vi "GetTraceFormat.vi"(8 "Error In":errorcluster, 11 "Keithley 6482 In":refnum<visa-resource-name>) -> (0 "Error Out":errorcluster, 2 "Trace Format Elements":T1[](array[typedef]), 3 "Keithley 6482 Out":refnum<visa-resource-name>)   [LabVIEW 8.6, in "Keithley-6482-Visa.lvlib"]
uses:
  Keithley-6482-Visa.lvlib
  Controls/TraceFormatElement.ctl
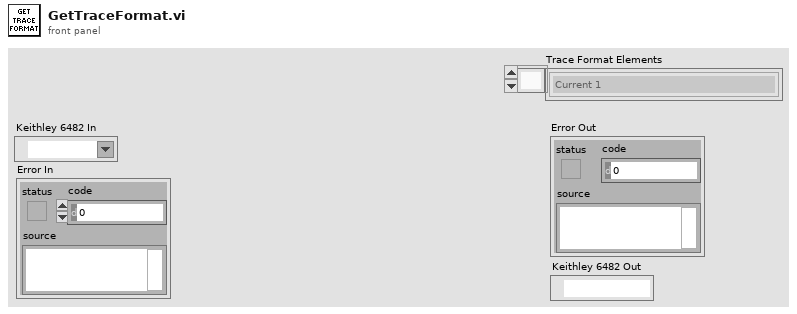
[diagram p1: front panel]
types:
  T1 = typedef "Keithley-6482-Visa.lvlib/TraceFormatElement.ctl" = enum16{"Current 1", "Current 2", "Calculate 1", "Calculate 2", "Calculate 3", "Calculate 4", "Calculate 5", "Calculate 6", "Calculate 7", "Time", "Status", "All", "Default"}
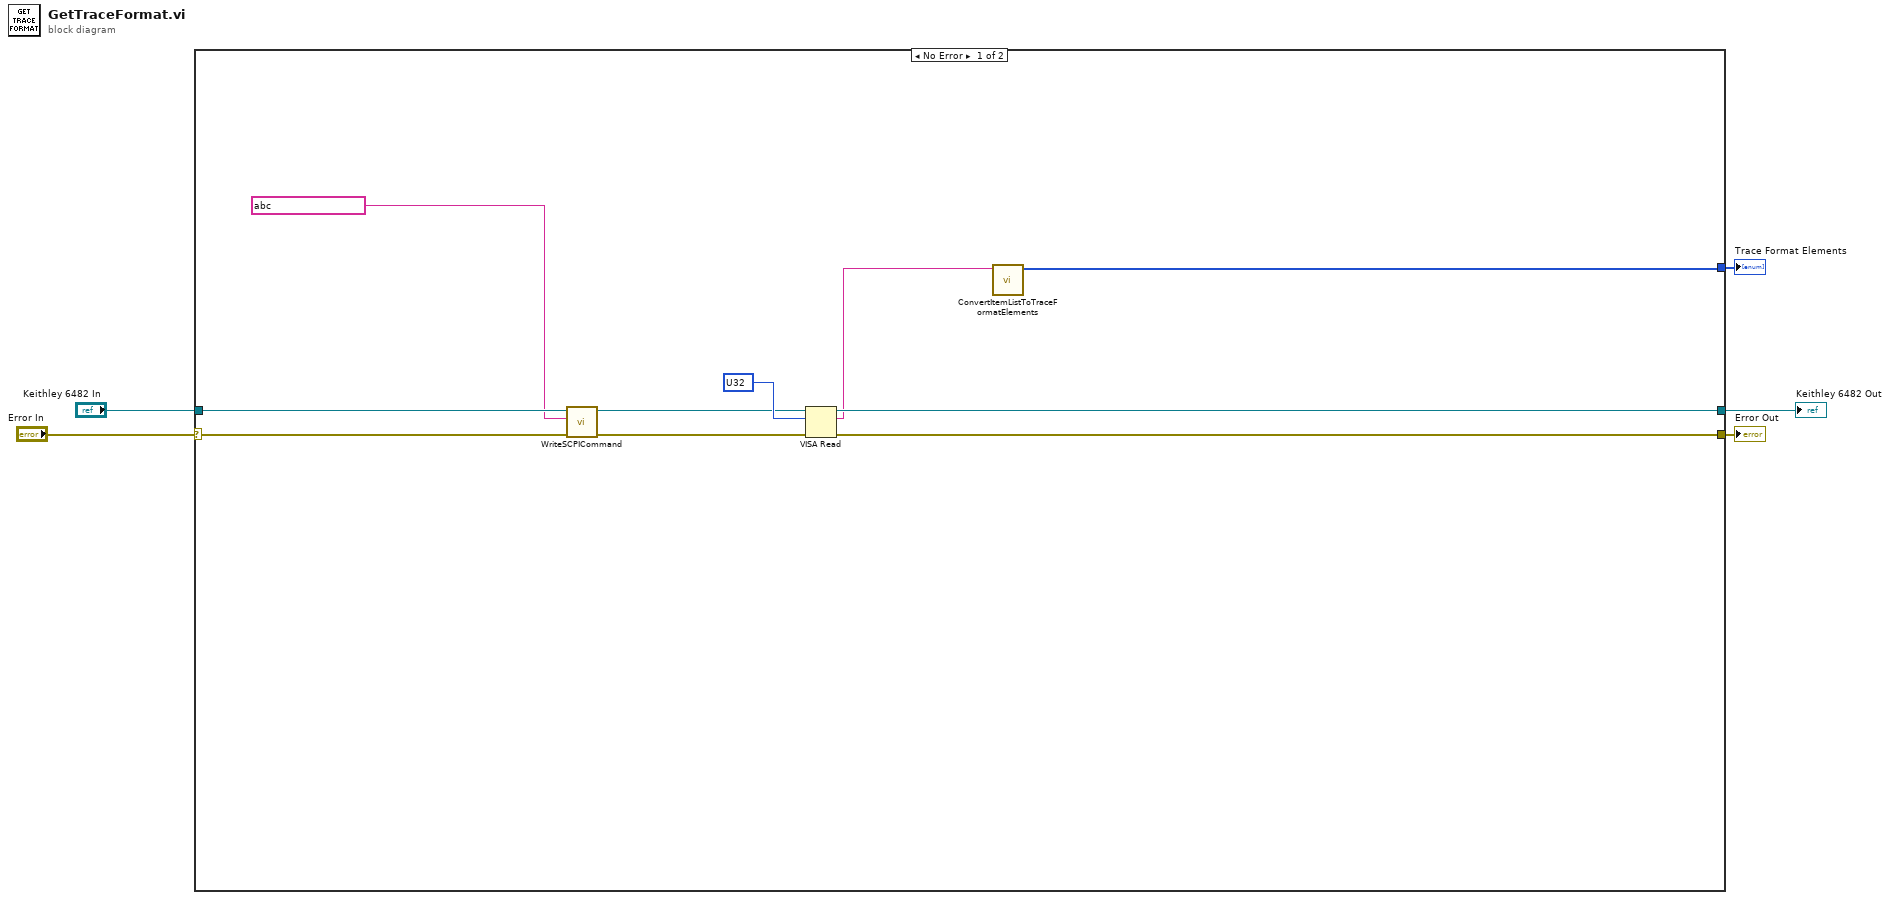
[diagram p0: block diagram]
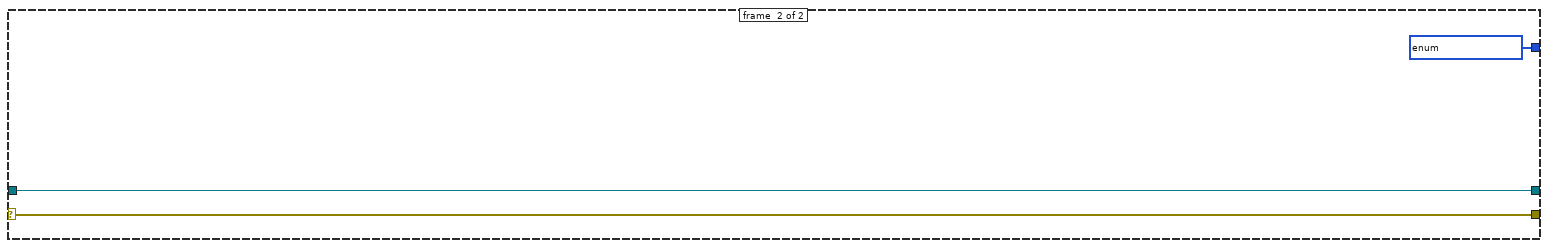
[diagram p2: hidden frame]
diagram:
  n1 = case shown="No Error" "Error In" {
    selector: "Error In" -> [w10 w17]
    tunnel: "Keithley 6482 In" -> [w9 w18]
    tunnel: [w15 w17] -> w3
    tunnel: [w14 w18] -> w2
    tunnel: [w6 w16] -> w1
    frame #0 {
      n2 = call "WriteSCPICommand.vi"("Error In"=w10, "SCPI Command"=string ?, "Keithley 6482 In"=w9) -> ("Error Out"=w11:errorcluster, "Keithley 6482 Out"=w12:refnum<visa-resource-name>)  [unwired: 7 in]
      n3 = VISA Read(VISA resource name=w12, byte count=u32 ?, error in (no error)=w11) -> (VISA resource name out=w14:refnum<visa-resource-name>, read buffer=w7:string, error out=w15:errorcluster)  [unwired: 1 out]
      n4 = call "ConvertItemListToTraceFormatElements.vi"("Item List"=w7) -> ("Trace Format Elements"=w6:T1[])  [unwired: 10 in]
    }
    frame #1 {
      w16 = T1[] ? items=["Current 1", "Current 2", "Calculate 1", "Calculate 2", "Calculate 3", "Calculate 4", "Calculate 5", "Calculate 6", "Calculate 7", "Time", "Status", "All", "Default"] ("Trace Format Elements")
    }
  }
  "Error Out" <- w3
  "Keithley 6482 Out" <- w2
  "Trace Format Elements" <- w1
